vi "BallShooter.vi"(8 "error in (no error)":errorcluster) -> (0 "error out":errorcluster)   [LabVIEW 2017]
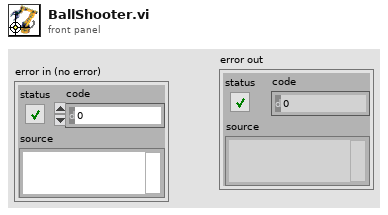
[diagram p1: front panel]
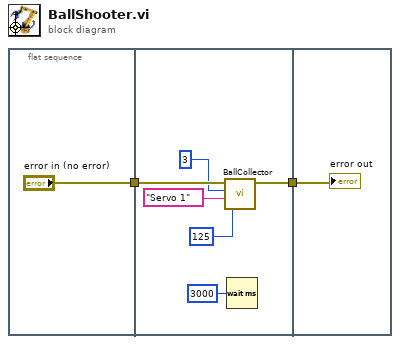
[diagram p0: block diagram]
diagram:
  n1 = flat-sequence {
    tunnel: ["error in (no error)"] -> w2
    tunnel: w2 -> [w9]
    tunnel: [w5] -> w1
    tunnel: w1 -> [w10]
    frame #0 {
    }
    frame #1 {
      n2 = call "BallCollector.vi"("Set Servo Position (0 - 180 degrees)"=u8 125, "Select Channel"="Servo 1", "Controller ID#  (I2C Address)"=u8 3, "Error/Flow In"=w9) -> ("Error/Flow Out"=w5:errorcluster)  [unwired: 3 in]
      n3 = Wait (ms)(milliseconds to wait=u32 3000) -> ()  [unwired: 1 out]
    }
    frame #2 {
      "error out" <- w10
    }
  }
